vi "ScaleTheValue.vi"(7 "physical channel":string, 8 "error in (no error)":errorcluster, 10 "Caps":T1, 11 "property":string) -> (0 "error out":errorcluster, 2 "dataType":string, 3 "offline value":variant)   [LabVIEW 2017]
uses:
  Ctrl/Caps.ctl
  Ctrl/Property.ctl
  Ctrl/PhysicalChannel.ctl
  Ctrl/Register.ctl
  Ctrl/Bitfield.ctl
  Ctrl/Scale.ctl
  Ctrl/ScaleType.ctl
  Ctrl/Enum.ctl
  Ctrl/EnumValue.ctl
  Ctrl/PolynomialScale.ctl
  Ctrl/LinearScale.ctl
  Ctrl/TableScale.ctl
  Ctrl/Coercion.ctl
  API/Bitfield/GetBitfiledValue(I32).vi
  API/Bitfield/GetBitfiledValue(U32).vi
  API/Bitfield/GetBitfiledValue(I64).vi
  API/Bitfield/GetBitfiledValue(U64).vi
  API/Bitfield/GetBitfiledValue(Bool).vi
  API/Bitfield/GetBitfiledValue(DBL).vi
  API/Scale/Scale(Polynomial).vi
  API/Scale/Scale(Linear).vi
  API/Scale/Scale(Table).vi
  API/Bitfield/Bitfield.lvlib
  <vilib>/Utility/Data Type/NI_Data Type.lvlib
  API/Scale/Scale.lvlib
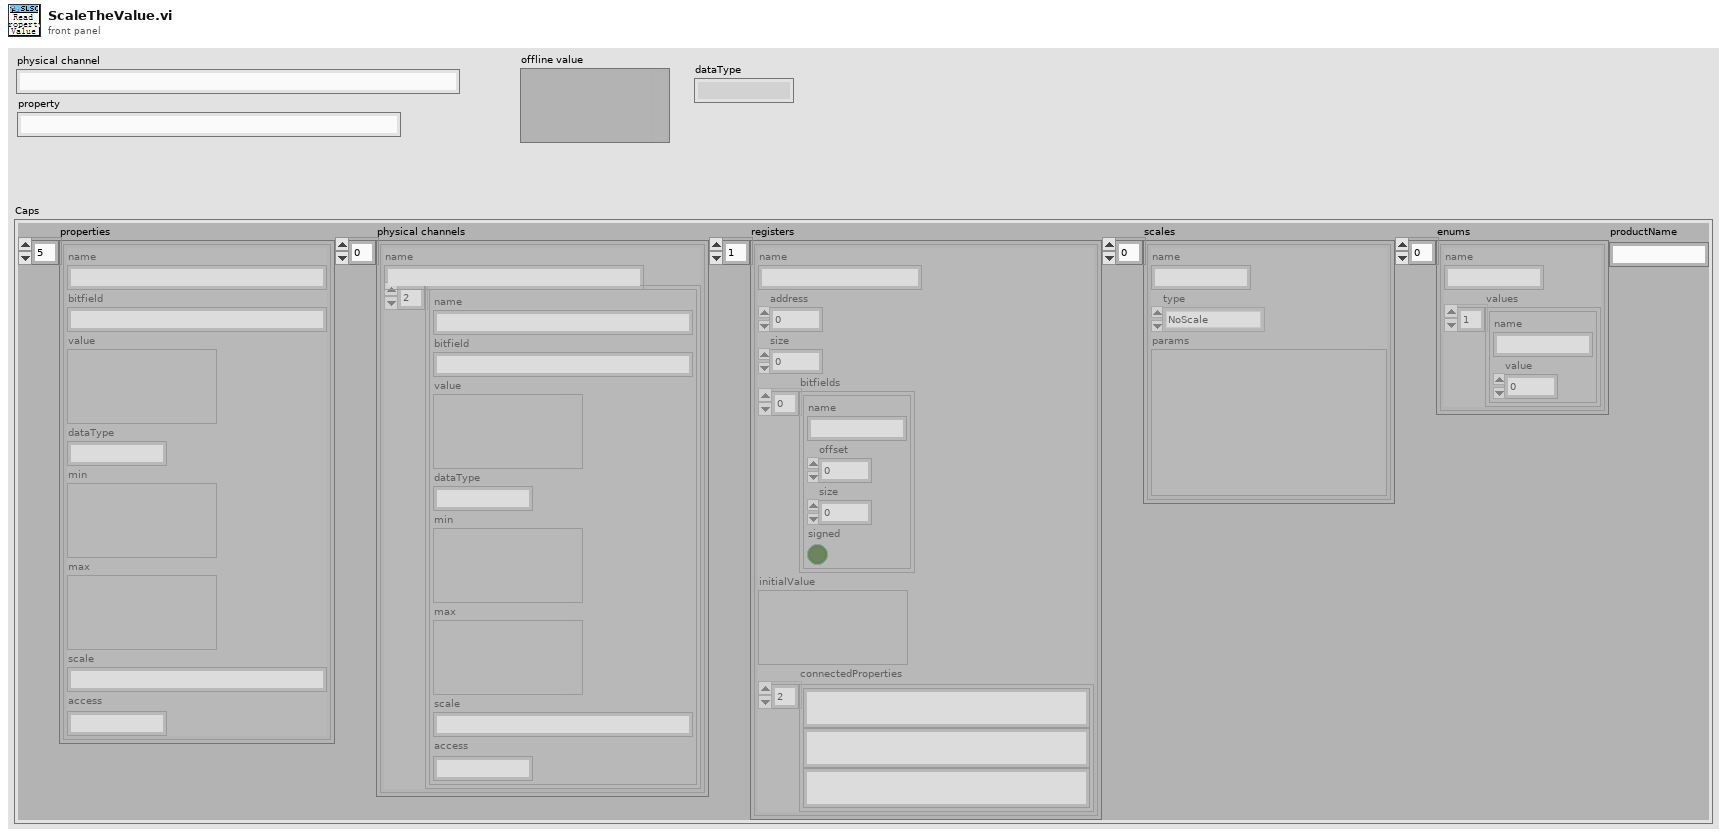
[diagram p1: front panel]
types:
  T1 = typedef "Caps.ctl" = cluster{"properties":T2[], "physical channels":T3[], "registers":T4[], "scales":T6[], "enums":T8[], "productName":string}
  T2 = typedef "Property.ctl" = cluster{"name":string, "bitfield":string, "value":variant, "dataType":string, "min":variant, "max":variant, "scale":string, "access":string}
  T3 = typedef "PhysicalChannel.ctl" = cluster{"name":string, "properties":T2[]}
  T4 = typedef "Register.ctl" = cluster{"name":string, "address":i32, "size":i32, "bitfields":T5[], "initialValue":variant, "connectedProperties":string[]}
  T5 = typedef "Bitfield.ctl" = cluster{"name":string, "offset":i32, "size":i32, "signed":bool}
  T6 = typedef "Scale.ctl" = cluster{"name":string, "type":T7, "params":variant}
  T7 = typedef "ScaleType.ctl" = enum16{"NoScale", "Table", "Polynomial", "Linear"}
  T8 = typedef "Enum.ctl" = cluster{"name":string, "values":T9[]}
  T9 = typedef "EnumValue.ctl" = cluster{"name":string, "value":i32}
  T10 = cluster{"Property":T2, "register":T4, "bitfield":T5, "scale":T6, "enum":T8}
  T11 = typedef "PolynomialScale.ctl" = cluster{"name":string, "forwardCoeffs":dbl[], "reverseCoeffs":dbl[]}
  T12 = typedef "LinearScale.ctl" = cluster{"name":string, "m":dbl, "b":dbl}
  T13 = typedef "TableScale.ctl" = cluster{"name":string, "coercion":string, "table":cluster{"scaled":dbl, "unscaled":dbl}[]}
  T14 = typedef "Coercion.ctl" = enum16{"Strict", "RoundToNearest", "Interpolate"}
  T15 = typedef "NI_Data Type.lvlib/Data Type.ctl" = enum8{"Invalid Type", "Void", "I8", "I16", "I32", "I64", "U8", "U16", "U32", "U64", "Single Float", "Double Float", "Extended Float", "Single Complex", "Double Complex", "Extended Complex", "Enum U8", "Enum U16", "Enum U32", "Enum U64", "Single Float With Unit", "Double Float With Unit", "Extended Float With Unit", "Single Complex with Unit", "Double Complex with Unit", "Extended Complex with Unit", "Boolean", "String", "Path", "Picture", "Tag", "Array", "Cluster", "Variant", "LV Variant", "Waveform", "Timestamp", "Digital Waveform", "Digital Data", "ExpressData", "Refnum", "External Data", "VI", "Poly VI", "LabVIEW Class Instance", "Fixed Point"}
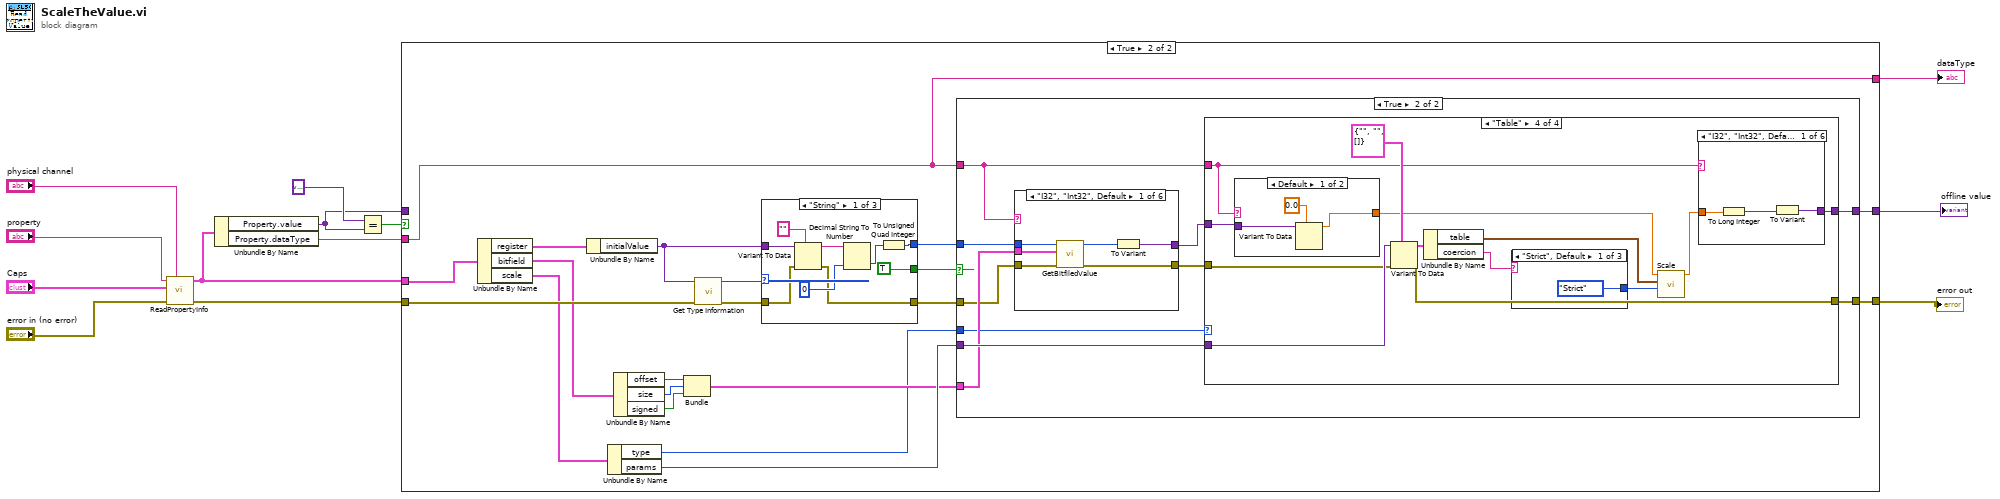
[diagram p0: block diagram]
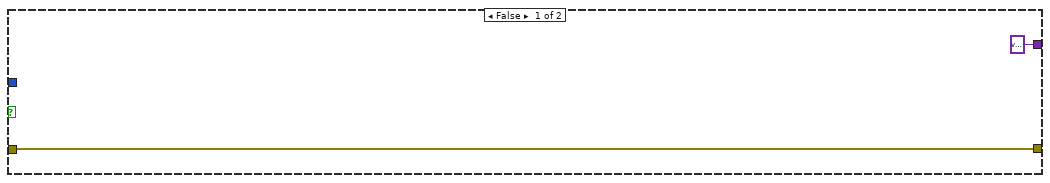
[diagram p3: hidden frame]
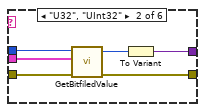
[diagram p4: hidden frame]
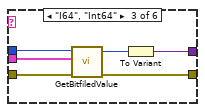
[diagram p5: hidden frame]
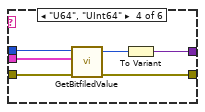
[diagram p6: hidden frame]
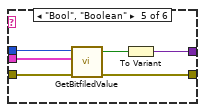
[diagram p7: hidden frame]
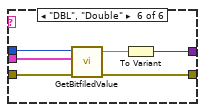
[diagram p8: hidden frame]
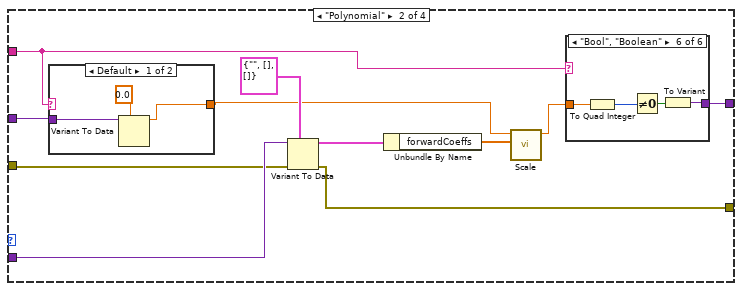
[diagram p10: hidden frame]
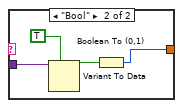
[diagram p11: hidden frame]
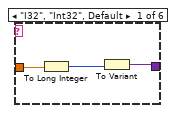
[diagram p12: hidden frame]
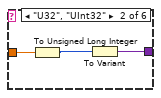
[diagram p13: hidden frame]
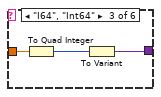
[diagram p14: hidden frame]
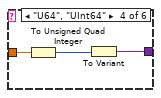
[diagram p15: hidden frame]
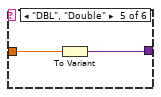
[diagram p16: hidden frame]
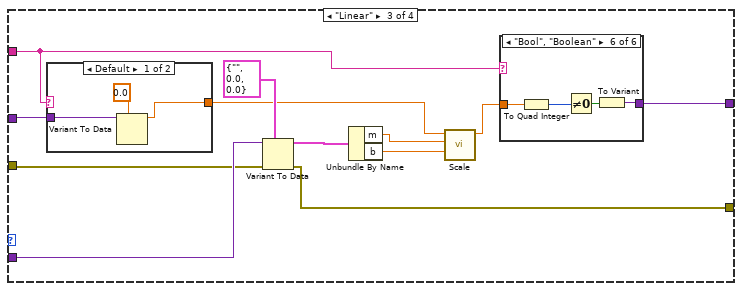
[diagram p17: hidden frame]
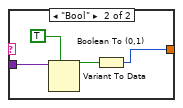
[diagram p18: hidden frame]
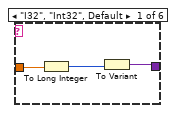
[diagram p19: hidden frame]
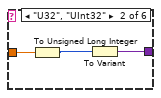
[diagram p20: hidden frame]
diagram:
  n1 = call "ReadPropertyInfo.vi"("physical channel"="physical channel", "error in (no error)"="error in (no error)", "Caps"="Caps", "property"="property") -> ("error out"=w12:errorcluster, "property info"=w11:T10)  [unwired: 6 in]
  n2 = Unbundle By Name(w11) -> ("Property.value"=w8:variant, "Property.dataType"=w2:string)
  n3 = Equal?(x=variant, y=w8) -> (x = y?=w9:bool)
  n4 = case shown="True" w9 {
    tunnel: w11 -> [_ w36]
    tunnel: [w16 w35] -> w3
    tunnel: [w15 w34] -> w13
    tunnel: [w14 w18] -> w4
    tunnel: w12 -> [w16 w33]
    tunnel: w2 -> [w14 w18]
    tunnel: w8 -> [w15 _]
    frame False {
    }
    frame True {
      n5 = Unbundle By Name(w36) -> ("register"=w32:T4, "bitfield"=w31:T5, "scale"=w30:T6)
      n6 = Unbundle By Name(w32) -> ("initialValue"=w26:variant)
      n7 = Unbundle By Name(w30) -> ("type"=w19:T7, "params"=w25:variant)
      n8 = Unbundle By Name(w31) -> ("offset"=w29:i32, "size"=w23:i32, "signed"=w24:bool)
      n9 = Bundle("offset"=w29, "size"=w23, "signed"=w24) -> (w21:cluster{"offset":i32, "size":i32, "signed":bool})  [unwired: 1 in]
      n10 = call <vilib>:"Get Type Information.vi"("error in (no error)"=w33, "Variant"=w26) -> ("error out"=w22:errorcluster, "Type"=w27:T15)  [unwired: 5 in, 3 out]
      n11 = case shown="\"String\"" w27 {
        tunnel: [w207 w214 u64 0] -> w28
        tunnel: w26 -> [w204 w211 _]
        tunnel: w22 -> [w203 w213 w217]
        tunnel: [w202 w212 w217] -> w20
        tunnel: [TRUE TRUE FALSE] -> w17
        frame "String" {
          n12 = Variant To Data(error in=w203, type="", Variant=w204) -> (data=w208:string, error out=w202:errorcluster)
          n13 = Decimal String To Number(string=w208, default (0L)=u64 0 ("default (0 I32)")) -> (number=w206:u64)  [unwired: 1 in, 1 out]
          n14 = To Unsigned Quad Integer(1:w206) -> (0:w207:u64)
        }
        frame "U64" {
          n15 = Variant To Data(error in=w213, type=u64 0, Variant=w211) -> (data=w214:u64, error out=w212:errorcluster)
        }
        frame Default {
          # "Not Specified"
        }
      }
      n16 = case shown="True" w17 {
        tunnel: [w37 w48] -> w35
        tunnel: [variant ("Variant") w47] -> w34
        tunnel: w28 -> [_ w46]
        tunnel: w25 -> [_ w45]
        tunnel: w21 -> [_ w44]
        tunnel: w20 -> [w37 w43]
        tunnel: w19 -> [_ w42]
        tunnel: w18 -> [_ w39]
        frame False {
        }
        frame True {
          n17 = case shown="\"I32\", \"Int32\", Default" w39 {
            tunnel: w46 -> [w54 w60 w66 w72 w78 w84]
            tunnel: w44 -> [w53 w59 w65 w71 w77 w83]
            tunnel: w43 -> [w51 w58 w64 w70 w76 w82]
            tunnel: [w50 w57 w63 w69 w75 w81] -> w41
            tunnel: [w49 w55 w61 w67 w73 w79] -> w40
            frame "I32", "Int32", Default {
              n18 = call-poly "GetBitfiledValue.vi"("error in"=w51, "bitfield caps"=w53, "register value"=w54) -> ("error out"=w50:errorcluster, "bitfield balue"=w52:i32)  [unwired: 7 in]
              n19 = To Variant(anything=w52) -> (Variant=w49:variant)
            }
            frame "U32", "UInt32" {
              n20 = call-poly "GetBitfiledValue.vi"("error in"=w58, "bitfield caps"=w59, "register value"=w60) -> ("error out"=w57:errorcluster, "bitfield balue"=w56:u32)  [unwired: 7 in]
              n21 = To Variant(anything=w56) -> (Variant=w55:variant)
            }
            frame "I64", "Int64" {
              n22 = call-poly "GetBitfiledValue.vi"("error in"=w64, "bitfield caps"=w65, "register value"=w66) -> ("error out"=w63:errorcluster, "bitfield balue"=w62:i64)  [unwired: 7 in]
              n23 = To Variant(anything=w62) -> (Variant=w61:variant)
            }
            frame "U64", "UInt64" {
              n24 = call-poly "GetBitfiledValue.vi"("error in"=w70, "bitfield caps"=w71, "register value"=w72) -> ("error out"=w69:errorcluster, "bitfield balue"=w68:u64)  [unwired: 7 in]
              n25 = To Variant(anything=w68) -> (Variant=w67:variant)
            }
            frame "Bool", "Boolean" {
              n26 = call-poly "GetBitfiledValue.vi"("error in"=w76, "bitfield caps"=w77, "register value"=w78) -> ("error out"=w75:errorcluster, "bitfield balue"=w74:bool)  [unwired: 7 in]
              n27 = To Variant(anything=w74) -> (Variant=w73:variant)
            }
            frame "DBL", "Double" {
              n28 = call-poly "GetBitfiledValue.vi"("error in"=w82, "bitfield caps"=w83, "register value"=w84) -> ("error out"=w81:errorcluster, "bitfield balue"=w80:dbl)  [unwired: 7 in]
              n29 = To Variant(anything=w80) -> (Variant=w79:variant)
            }
          }
          n30 = case shown="\"Table\"" w42 {
            tunnel: w45 -> [_ w94 w132 w170]
            tunnel: w41 -> [w85 w93 w131 w169]
            tunnel: w40 -> [w86 w88 w124 w161]
            tunnel: [w85 w92 w130 w163] -> w48
            tunnel: w39 -> [_ w87 w125 w162]
            tunnel: [w86 w90 w128 w167] -> w47
            frame "NoScale", Default {
            }
            frame "Polynomial" {
              n31 = case shown="Default" w87 {
                tunnel: w88 -> [w100 w103]
                tunnel: [w98 w101] -> w89
                frame Default {
                  n32 = Variant To Data(type=0.0 ("unscaled value"), Variant=w100) -> (data=w98:dbl)  [unwired: 1 in, 1 out]
                }
                frame "Bool" {
                  n33 = Variant To Data(type=TRUE, Variant=w103) -> (data=w102:bool)  [unwired: 1 in, 1 out]
                  n34 = Boolean To (0,1)(Boolean=w102) -> (0, 1=w101:i16)
                }
              }
              n35 = Variant To Data(error in=w93, type=T11 {"name"="", "forwardCoeffs"=[], "reverseCoeffs"=[]} ("PolynomialScale"), Variant=w94) -> (data=w97:T11, error out=w92:errorcluster)
              n36 = Unbundle By Name(w97) -> ("forwardCoeffs"=w95:dbl[])
              n37 = call-poly "Scale.vi"("forward coeffs"=w95, "unscaled value"=w89) -> ("scale value"=w91:dbl)  [unwired: 9 in]
              n38 = case shown="\"Bool\", \"Boolean\"" w87 {
                tunnel: w91 -> [w106 w110 w113 w115 w118 w122]
                tunnel: [w105 w108 w111 w114 w117 w119] -> w90
                frame "I32", "Int32", Default {
                  n39 = To Long Integer(number=w106) -> (32bit integer=w107:i32)
                  n40 = To Variant(anything=w107) -> (Variant=w105:variant)
                }
                frame "U32", "UInt32" {
                  n41 = To Unsigned Long Integer(number=w110) -> (unsigned 32bit integer=w109:u32)
                  n42 = To Variant(anything=w109) -> (Variant=w108:variant)
                }
                frame "I64", "Int64" {
                  n43 = To Quad Integer(1:w113) -> (0:w112:i64)
                  n44 = To Variant(anything=w112) -> (Variant=w111:variant)
                }
                frame "U64", "UInt64" {
                  n45 = To Unsigned Quad Integer(1:w115) -> (0:w116:u64)
                  n46 = To Variant(anything=w116) -> (Variant=w114:variant)
                }
                frame "DBL", "Double" {
                  n47 = To Variant(anything=w118) -> (Variant=w117:variant)
                }
                frame "Bool", "Boolean" {
                  n48 = To Quad Integer(1:w122) -> (0:w121:i64)
                  n49 = Not Equal To 0?(x=w121) -> (x != 0?=w120:bool)
                  n50 = To Variant(anything=w120) -> (Variant=w119:variant)
                }
              }
            }
            frame "Linear" {
              n51 = case shown="Default" w125 {
                tunnel: w124 -> [w137 w140]
                tunnel: [w135 w138] -> w123
                frame Default {
                  n52 = Variant To Data(type=0.0 ("unscaled value"), Variant=w137) -> (data=w135:dbl)  [unwired: 1 in, 1 out]
                }
                frame "Bool" {
                  n53 = Variant To Data(type=TRUE, Variant=w140) -> (data=w139:bool)  [unwired: 1 in, 1 out]
                  n54 = Boolean To (0,1)(Boolean=w139) -> (0, 1=w138:i16)
                }
              }
              n55 = Variant To Data(error in=w131, type=T12 {"name"="", "m"=0.0, "b"=0.0} ("LinearScale"), Variant=w132) -> (data=w134:T12, error out=w130:errorcluster)
              n56 = Unbundle By Name(w134) -> ("m"=w127:dbl, "b"=w126:dbl)
              n57 = call-poly "Scale.vi"("offset"=w126, "multiplier"=w127, "unscaled value"=w123) -> ("scaled value"=w129:dbl)  [unwired: 8 in]
              n58 = case shown="\"Bool\", \"Boolean\"" w125 {
                tunnel: w129 -> [w143 w147 w150 w152 w155 w159]
                tunnel: [w142 w145 w148 w151 w154 w156] -> w128
                frame "I32", "Int32", Default {
                  n59 = To Long Integer(number=w143) -> (32bit integer=w144:i32)
                  n60 = To Variant(anything=w144) -> (Variant=w142:variant)
                }
                frame "U32", "UInt32" {
                  n61 = To Unsigned Long Integer(number=w147) -> (unsigned 32bit integer=w146:u32)
                  n62 = To Variant(anything=w146) -> (Variant=w145:variant)
                }
                frame "I64", "Int64" {
                  n63 = To Quad Integer(1:w150) -> (0:w149:i64)
                  n64 = To Variant(anything=w149) -> (Variant=w148:variant)
                }
                frame "U64", "UInt64" {
                  n65 = To Unsigned Quad Integer(1:w152) -> (0:w153:u64)
                  n66 = To Variant(anything=w153) -> (Variant=w151:variant)
                }
                frame "DBL", "Double" {
                  n67 = To Variant(anything=w155) -> (Variant=w154:variant)
                }
                frame "Bool", "Boolean" {
                  n68 = To Quad Integer(1:w159) -> (0:w158:i64)
                  n69 = Not Equal To 0?(x=w158) -> (x != 0?=w157:bool)
                  n70 = To Variant(anything=w157) -> (Variant=w156:variant)
                }
              }
            }
            frame "Table" {
              n71 = case shown="Default" w162 {
                tunnel: w161 -> [w175 w178]
                tunnel: [w173 w176] -> w160
                frame Default {
                  n72 = Variant To Data(type=0.0 ("unscaled value"), Variant=w175) -> (data=w173:dbl)  [unwired: 1 in, 1 out]
                }
                frame "Bool" {
                  n73 = Variant To Data(type=TRUE, Variant=w178) -> (data=w177:bool)  [unwired: 1 in, 1 out]
                  n74 = Boolean To (0,1)(Boolean=w177) -> (0, 1=w176:i16)
                }
              }
              n75 = Variant To Data(error in=w169, type=T13 {"name"="", "coercion"="", "table"=[]} ("TableScale"), Variant=w170) -> (data=w172:T13, error out=w163:errorcluster)
              n76 = Unbundle By Name(w172) -> ("table"=w166:cluster{"scaled":dbl, "unscaled":dbl}[], "coercion"=w165:string)
              n77 = case shown="\"Strict\", Default" w165 {
                tunnel: [Coercion."Strict" ("coercion") Coercion."RoundToNearest" ("coercion") Coercion."Interpolate" ("coercion")] -> w164
                frame "Strict", Default {
                }
                frame "RoundToNearest" {
                }
                frame "Interpolate" {
                }
              }
              n78 = call-poly "Scale.vi"("coercion"=w164, "scales"=w166, "unscaled value"=w160) -> ("scaled value"=w168:dbl)  [unwired: 8 in]
              n79 = case shown="\"I32\", \"Int32\", Default" w162 {
                tunnel: w168 -> [w184 w188 w191 w193 w196 w200]
                tunnel: [w183 w186 w189 w192 w195 w197] -> w167
                frame "I32", "Int32", Default {
                  n80 = To Long Integer(number=w184) -> (32bit integer=w185:i32)
                  n81 = To Variant(anything=w185) -> (Variant=w183:variant)
                }
                frame "U32", "UInt32" {
                  n82 = To Unsigned Long Integer(number=w188) -> (unsigned 32bit integer=w187:u32)
                  n83 = To Variant(anything=w187) -> (Variant=w186:variant)
                }
                frame "I64", "Int64" {
                  n84 = To Quad Integer(1:w191) -> (0:w190:i64)
                  n85 = To Variant(anything=w190) -> (Variant=w189:variant)
                }
                frame "U64", "UInt64" {
                  n86 = To Unsigned Quad Integer(1:w193) -> (0:w194:u64)
                  n87 = To Variant(anything=w194) -> (Variant=w192:variant)
                }
                frame "DBL", "Double" {
                  n88 = To Variant(anything=w196) -> (Variant=w195:variant)
                }
                frame "Bool", "Boolean" {
                  n89 = To Quad Integer(1:w200) -> (0:w199:i64)
                  n90 = Not Equal To 0?(x=w199) -> (x != 0?=w198:bool)
                  n91 = To Variant(anything=w198) -> (Variant=w197:variant)
                }
              }
            }
          }
        }
      }
    }
  }
  "offline value" <- w13
  "error out" <- w3
  "dataType" <- w4
